vi "QueueStatus.vi"(8 "error in (no error)":errorcluster, 10 "Return Elements? (F)":bool, 11 "MessageQueue in":refnum<class "MessageQueue.lvclass">) -> (0 "error out":errorcluster, 1 "# Pending Insert":i32, 2 "# Pending Remove":i32, 3 "MessageQueue out":refnum<class "MessageQueue.lvclass">, 4 "# Message in Queue":i32, 5 "Queue Name":string, 6 "Messages":refnum<class "Message.lvclass">[](array[class]), 7 "Max Queue Size":i32)   [LabVIEW 2009, in "LapDog.Messaging.v2.lvlib" / "MessageQueue.lvclass"]
doc: "Returns information about the state of the queue. This vi can be used to test if the queue is valid. Invalid queues return error 1."
uses:
  MessageQueue.lvclass
  MessageObject/Message.lvclass
  MessageQueue.lvclass/MessageQueue.ctl
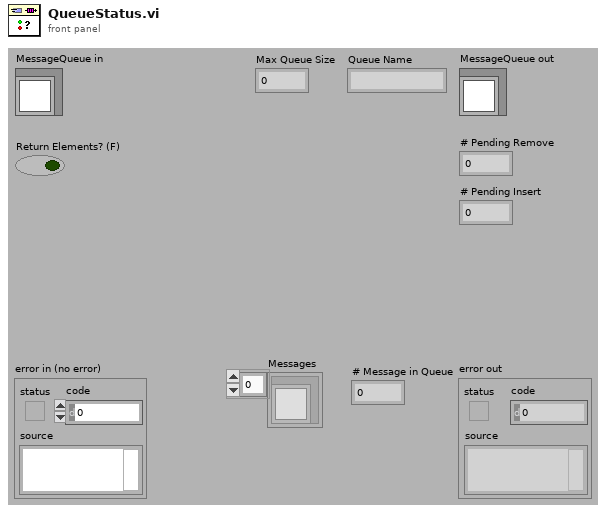
[diagram p1: front panel]
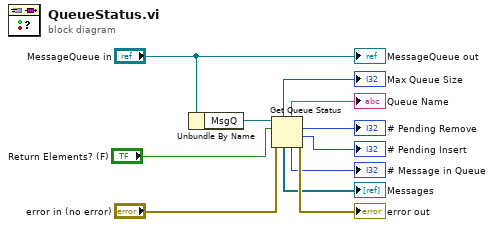
[diagram p0: block diagram]
diagram:
  n1 = Unbundle By Name("MessageQueue in") -> ("MsgQ"=w10:refnum<queue>)
  n2 = Get Queue Status(queue=w10, return elements? (F)="Return Elements? (F)", error in (no error)="error in (no error)") -> (queue name=→"Queue Name":string, max queue size=→"Max Queue Size":i32, # pending remove=→"# Pending Remove":i32, # pending insert=→"# Pending Insert":i32, error out=→"error out":errorcluster, # elements in queue=→"# Message in Queue":i32, elements=→"Messages":refnum<class "Message.lvclass">[])  [unwired: 1 out]
  "MessageQueue out" <- "MessageQueue in"
